vi "DDS RAM Enable.vi"(6 "channel number (1)":u8=1 min=1 max=4 step=1, 8 "error in":errorcluster, 9 "RAM Enable":bool, 10 "RAM Dest Type":u8, 11 "DDS ref in":T1={"NI USB-8451 device reference"="", "DIO port"=0, "Serial Clock Rate [kHz]"=1000}) -> (0 "error out":errorcluster, 3 "DDS ref out":T1={"NI USB-8451 device reference"="", "DIO port"=0, "Serial Clock Rate [kHz]"=1000})   [LabVIEW 2013]
doc: "This VI will enable or disable the RAM bit as appropriate and also programs the correct values into the RAM destination bits."
uses:
  DDS_box_device_reference.ctl
  <vilib>/ni845x/ni845x.llb/ni845xControl.ctl
  AD9910 registers.ctl
panel:
  out "CFR1":u8[](array[numeric])
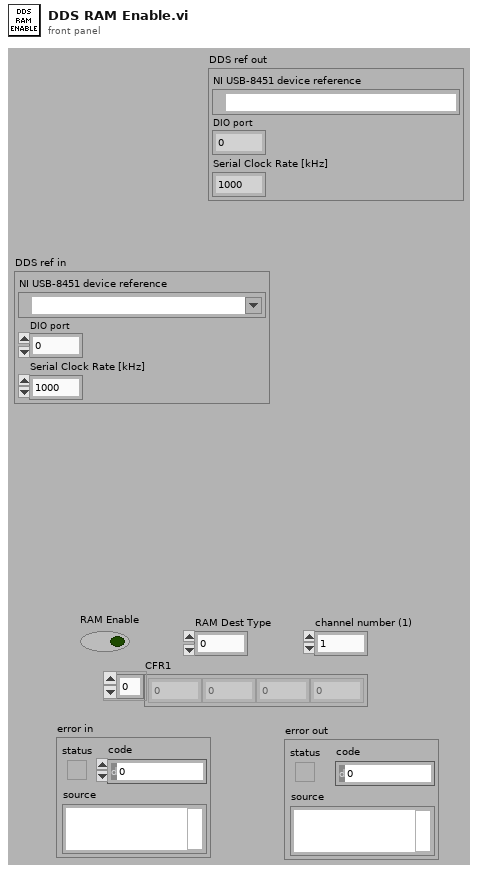
[diagram p1: front panel]
types:
  T1 = typedef "DDS_box_device_reference.ctl" = cluster{"NI USB-8451 device reference":T2, "DIO port":u8, "Serial Clock Rate [kHz]":u16}
  T2 = typedef "ni845xControl.ctl" = refnum<k21>
  T3 = typedef "AD9910 registers.ctl" = enum16{"CFR1", "CFR2", "CFR3", "Auxiliary DAC Control", "I/0 Update Rate", "Frequency Tuning Word", "Phase Offset Word", "Amplitude Scale Factor", "Multichip Sync", "Digital Ramp Limit", "Digital Ramp Step Size", "Digital Ramp Rate", "Single Tone Profile 0", "Single Tone Profile 1", "Single Tone Profile 2", "Single Tone Profile 3", "Single Tone Profile 4", "Single Tone Profile 5", "Single Tone Profile 6", "Single Tone Profile 7", "RAM Profile 0", "RAM Profile 1", "RAM Profile 2", "RAM Profile 3", "RAM Profile 4", "RAM Profile 5", "RAM Profile 6", "RAM Profile 7", "RAM"}
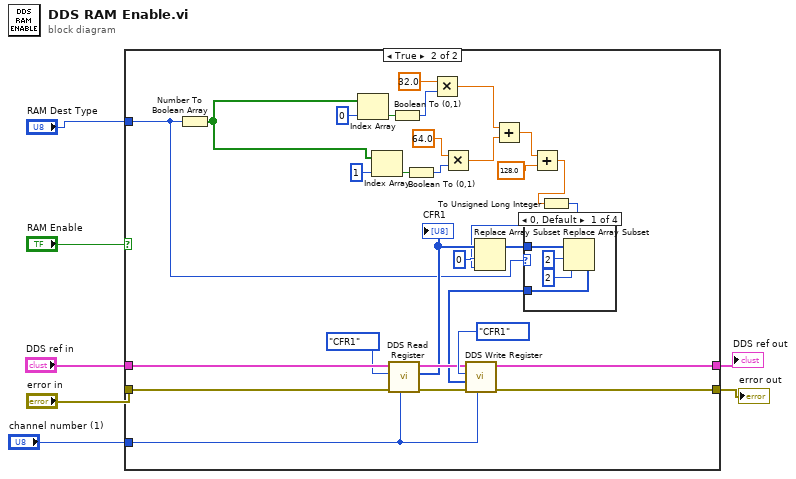
[diagram p0: block diagram]
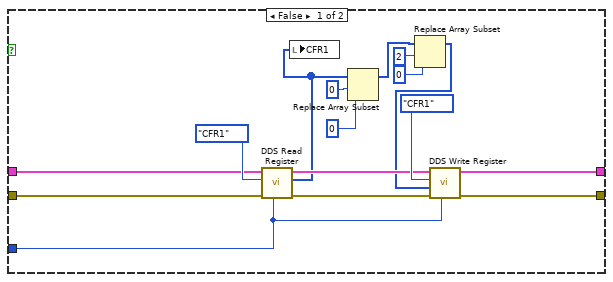
[diagram p2: hidden frame]
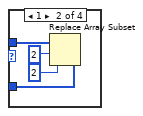
[diagram p3: hidden frame]
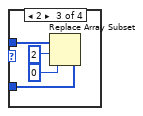
[diagram p4: hidden frame]
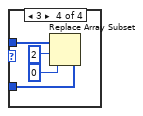
[diagram p5: hidden frame]
diagram:
  n1 = case shown="True" "RAM Enable" {
    tunnel: [w23 w52] -> w3
    tunnel: [w22 w51] -> w4
    tunnel: "DDS ref in" -> [w18 w49]
    tunnel: "error in" -> [w17 w48]
    tunnel: "channel number (1)" -> [w12 w27]
    tunnel: "RAM Dest Type" -> [_ w24]
    frame False {
      n2 = call "DDS Read Register.vi"("channel number (1)"=w12, "error in (no error)"=w17, "Register"=AD9910_registers."CFR1", "DDS ref in"=w18) -> ("error out"=w14:errorcluster, "Read data"=w13:u8[], "DDS ref out"=w15:T1)  [unwired: 5 in]
      n3 = local write "CFR1"(w13) -> ()
      n4 = Replace Array Subset(array=w13, new element=u8 0 ("new element/subarray"), index=0) -> (w9:u8[])
      n5 = Replace Array Subset(array=w9, new element=u8 0 ("new element/subarray"), index=2) -> (w8:u8[])
      n6 = call "DDS Write Register.vi"("channel number (1)"=w12, "error in (no error)"=w14, "Write Data"=w8, "Register"=AD9910_registers."CFR1", "DDS ref in"=w15) -> ("error out"=w22:errorcluster, "DDS ref out"=w23:T1)  [unwired: 5 in]
    }
    frame True {
      n7 = Number To Boolean Array(number=w24) -> (Boolean array=w36:bool[])
      n8 = Index Array(array=w36, index=0) -> (element=w40:bool)
      n9 = Index Array(array=w36, index=1) -> (element=w37:bool)
      n10 = call "DDS Read Register.vi"("channel number (1)"=w27, "error in (no error)"=w48, "Register"=AD9910_registers."CFR1", "DDS ref in"=w49) -> ("error out"=w47:errorcluster, "Read data"=w44:u8[], "DDS ref out"=w46:T1)  [unwired: 5 in]
      "CFR1" <- w44
      n11 = Boolean To (0,1)(Boolean=w40) -> (0, 1=w39:i16)
      n12 = Boolean To (0,1)(Boolean=w37) -> (0, 1=w35:i16)
      n13 = Multiply(x=32.0, y=w39) -> (x*y=w33:dbl)
      n14 = Multiply(x=64.0, y=w35) -> (x*y=w32:dbl)
      n15 = Add(x=w33, y=w32) -> (x+y=w31:dbl)
      n16 = Add(x=w31, y=128.0) -> (x+y=w29:dbl)
      n17 = To Unsigned Long Integer(number=w29) -> (unsigned 32bit integer=w28:u32)
      n18 = Replace Array Subset(array=w44, new element=w28, index=0) -> (w26:u8[])
      n19 = case shown="0, Default" w24 {
        tunnel: w26 -> [w54 w59 w63 w67]
        tunnel: [w55 w58 w62 w66] -> w25
        frame 0, Default {
          n20 = Replace Array Subset(array=w54, new element=u8 2 ("new element/subarray"), index=2) -> (w55:u8[])
        }
        frame 1 {
          n21 = Replace Array Subset(array=w59, new element=u8 2 ("new element/subarray"), index=2) -> (w58:u8[])
        }
        frame 2 {
          n22 = Replace Array Subset(array=w63, new element=u8 0 ("new element/subarray"), index=2) -> (w62:u8[])
        }
        frame 3 {
          n23 = Replace Array Subset(array=w67, new element=u8 0 ("new element/subarray"), index=2) -> (w66:u8[])
        }
      }
      n24 = call "DDS Write Register.vi"("channel number (1)"=w27, "error in (no error)"=w47, "Write Data"=w25, "Register"=AD9910_registers."CFR1", "DDS ref in"=w46) -> ("error out"=w51:errorcluster, "DDS ref out"=w52:T1)  [unwired: 5 in]
    }
  }
  "error out" <- w4
  "DDS ref out" <- w3
